vi "testy 3dconnection.vi"(6 "axis info 2":T1, 8 "error in (no error)":errorcluster, 11 "SceneObject in":refnum<vi>) -> (3 "SceneObject out":refnum<vi>)   [LabVIEW 2015]
uses:
  <vilib>/picture/3D Picture Control/NI_3D Picture Control.lvlib
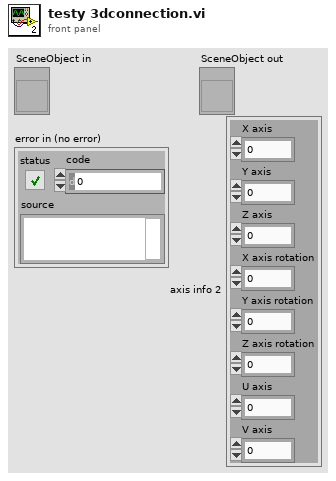
[diagram p1: front panel]
types:
  T1 = cluster{"X axis":i32, "Y axis":i32, "Z axis":i32, "X axis rotation":i32, "Y axis rotation":i32, "Z axis rotation":i32, "U axis":i32, "V axis":i32}
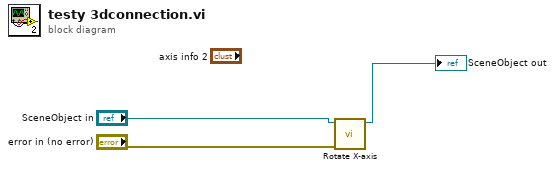
[diagram p0: block diagram]
diagram:
  n1 = call <vilib>:"Rotate X-axis.vi"("error in (no error)"="error in (no error)", "Scene Object In"="SceneObject in") -> ("Scene Object Out"=→"SceneObject out":refnum<vi>)  [unwired: 8 in, 1 out]
